vi "GetGraphChartReference.vi"(8 "error in":errorcluster, 11 "GraphChart in":refnum<class "GraphChart.lvclass">) -> (0 "error out":errorcluster, 1 "graph scale reference":refnum<vi>, 3 "GraphChart out":refnum<class "GraphChart.lvclass">)   [LabVIEW 2014, in "GraphChart.lvclass"]
uses:
  GraphChart.lvclass
  Generic/Generic.lvclass
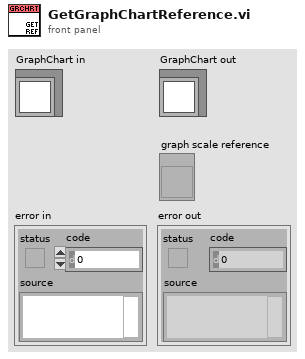
[diagram p1: front panel]
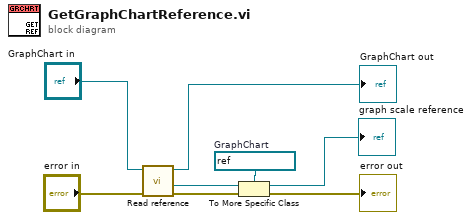
[diagram p0: block diagram]
diagram:
  w5 = refnum<vi> refnum  # GraphChart
  n1 = call "Read reference.vi"("error in"="error in", "GObject in"="GraphChart in") -> ("error out"=w6:errorcluster, "reference"=w7:refnum<vi>, "GObject out"=→"GraphChart out":refnum<class "GraphChart.lvclass">)  [unwired: 5 in]
  n2 = To More Specific Class(target class=w5, reference=w7, error in=w6) -> (specific class reference=→"graph scale reference":refnum<vi>, error out=→"error out":errorcluster)
